vi "String_Indicator (SubVI).vi"(11 "String in":refnum<vi>) -> ()   [LabVIEW 2017]
uses:
  Global_SNK3_HF.vi
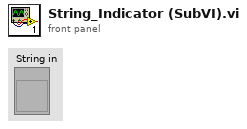
[diagram p1: front panel]
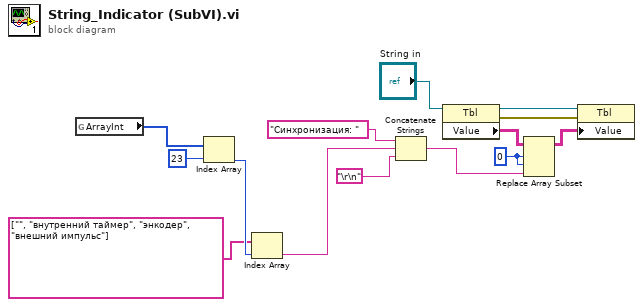
[diagram p0: block diagram]
diagram:
  w2 = 0 ("index (row)")
  n1 = global read "Global_SNK3_HF.vi" "ArrayInt"() -> (w7:i32[])
  n2 = Index Array(array=w7, index=23) -> (element=w10:i32)
  n3 = Index Array(array=string[] ["", "внутренний таймер", "энкодер", "внешний импульс"], index=w10) -> (element=w12:string)
  n4 = Concatenate Strings("Синхронизация: ", w12, "\r\n") -> (w1:string)
  n5 = property class="Tbl"(reference="String in") -> (reference out=w6:refnum<vi>, error out=w5:errorcluster, "Value"=w4:string[][])  [unwired: 1 in]
  n6 = Replace Array Subset(array=w4, new element=w1, index (row)=w2, index (col)=w2) -> (w3:string[][])
  n7 = property class="Tbl"(reference=w6, error in=w5, "Value"=w3) -> ()  [unwired: 2 out]
